vi "DeleteQ.vi"(8 "error in (no error)":errorcluster, 10 "QNames":string[](array[string])) -> (0 "error out":errorcluster, 1 "foundArray":bool[](array[boolean]))   [LabVIEW 2020, in "QDict.lvlib"]
doc: "Developed by Kevin Thompson\nkevin@thompsonengineering.net\n\nCopyright 2021\nThompson Engineering, LLC"
uses:
  QDict.lvlib
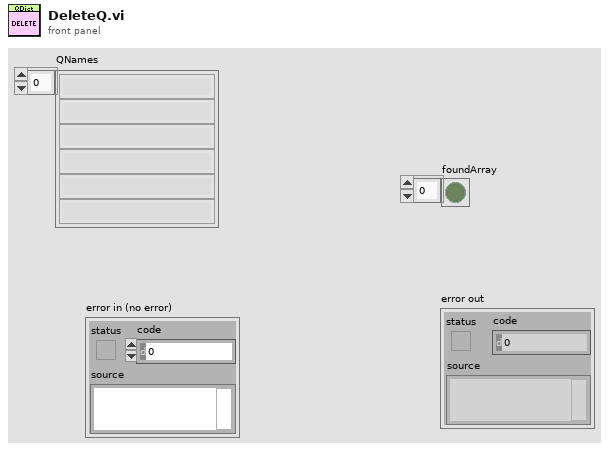
[diagram p1: front panel]
types:
  T1 = typedef "TD Dynamic CVT DVR--ref.ctl" = refnum<data-value>
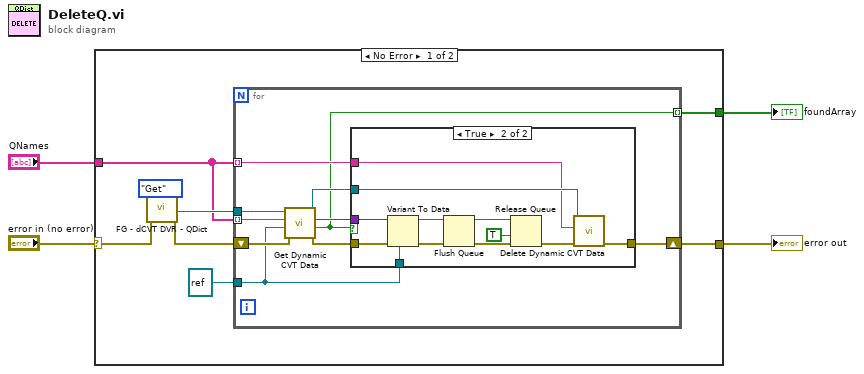
[diagram p0: block diagram]
diagram:
  n1 = case shown="No Error" "error in (no error)" {
    selector: "error in (no error)" -> [w11 w36]
    tunnel: [w6 w36] -> w4
    tunnel: "QNames" -> [w5 _]
    tunnel: [w7 _] -> w1
    frame No Error {
      n2 = call "FG - dCVT DVR - QDict.vi"("error in (no error)"=w11, "Action (Get)"=enum16{"Init", "Get", "Set"}."Get") -> ("dCVT QMH out"=w9:T1, "error out"=w10:errorcluster)  [unwired: 7 in]
      n3 = for {
        shift-right: [w15] -> w6
        shift-left: w10 -> [w20]
        tunnel: w9 -> [w22]
        tunnel: w5 -> [w21] mode=indexing
        tunnel: refnum<queue> refnum ("queue out") -> [w13]
        tunnel: [w14] -> w7 mode=indexing
        tunnel: w5 -> [w16] mode=indexing
        n4 = call <vilib>:"Get Dynamic CVT Data.vi"("error in (no error)"=w20, "default value (empty variant)"=w13, "DataName"=w21, "dCVT DVR"=w22) -> ("error out"=w19:errorcluster, "found"=w14:bool, "value"=w18:variant, "dCVT DVR out"=w17:T1)  [unwired: 4 in]
        n5 = case shown="True" w14 {
          tunnel: w19 -> [w23 w30]
          tunnel: w18 -> [_ w29]
          tunnel: w17 -> [_ w27]
          tunnel: w16 -> [_ w26]
          tunnel: [w23 w25] -> w15
          tunnel: w13 -> [_ w24]
          frame False {
          }
          frame True {
            n6 = Variant To Data(error in=w30, type=w24, Variant=w29) -> (data=w34:refnum<queue>, error out=w35:errorcluster)
            n7 = Flush Queue(queue=w34, error in (no error)=w35) -> (queue out=w32:refnum<queue>, error out=w33:errorcluster)  [unwired: 1 out]
            n8 = Release Queue(queue=w32, force destroy? (F)=TRUE, error in (no error)=w33) -> (error out=w28:errorcluster)  [unwired: 2 out]
            n9 = call <vilib>:"Delete Dynamic CVT Data.vi"("error in (no error)"=w28, "DataName"=w26, "dCVT DVR"=w27) -> ("error out"=w25:errorcluster)  [unwired: 6 in, 2 out]
          }
        }
      }
    }
    frame Error {
    }
  }
  "error out" <- w4
  "foundArray" <- w1
